vi "제목없음 2 (SubVI).vi"(9 "불리언":bool, 10 "문자열 입력":string, 11 "문자열":string) -> (3 "문자열 출력 2":string)   [LabVIEW 2018]
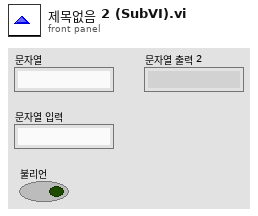
[diagram p1: front panel]
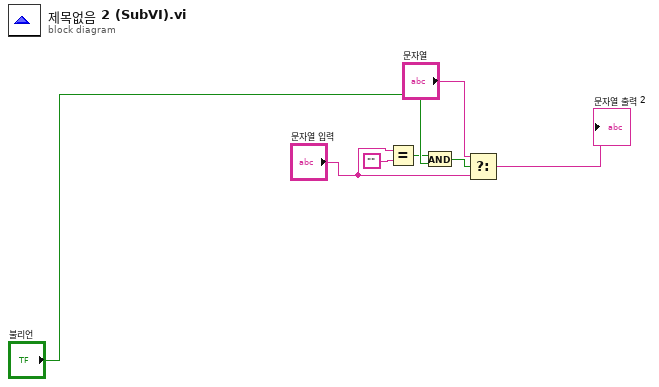
[diagram p0: block diagram]
diagram:
  n1 = Equal?(x="문자열 입력", y="") -> (x = y?=w2:bool)
  n2 = And(x=w2, y="불리언") -> (x .and. y?=w1:bool)
  n3 = Select(t="문자열", s=w1, f="문자열 입력") -> (s? t:f=→"문자열 출력 2":string)
